vi "Example_BP Network_Classification.vi"() -> ()   [LabVIEW 2020]
uses:
  <vilib>/addons/Machine Learning/Supervised Learning/ml_BP_Terminal Condition.ctl
  <vilib>/Utility/miscctls.llb/LV3DPointTypeDef.ctl
  <vilib>/addons/Machine Learning/Utilities/Training & Test Set (matrix-class).vi
  <vilib>/addons/Machine Learning/Visualization/Visualization (3D).vi
  <vilib>/addons/Machine Learning/NILabs_MLT.lvlib
panel:
  out "Test samples":i32
  in  "Test percentage":dbl
  in  "Num of samples":i32
  out "Lapsed time (ms)":i32
  in  "Data set":enum16{"4 Gaussians", "3 Concentric Circles"}(ring)
  out "Classification accuracy":dbl
  out "Test data":refnum<vi>(3d-picture)
  in  "Stopping criteria":T1={"min MSE"=1e-05, "min delta MSE"=1e-08, "min step length"=1e-08, "max iteration"=1000.0}
  in  "# of hidden neurons":i32=5
  out "Training data":refnum<vi>(3d-picture)
  out "Training MSE":dbl
  # "Introduction:\nA Back-propagation (BP) neural network is applied to two classification problems."
  # "%"
  # "(Samples are overlain with class labels predicted by the BP network.)"
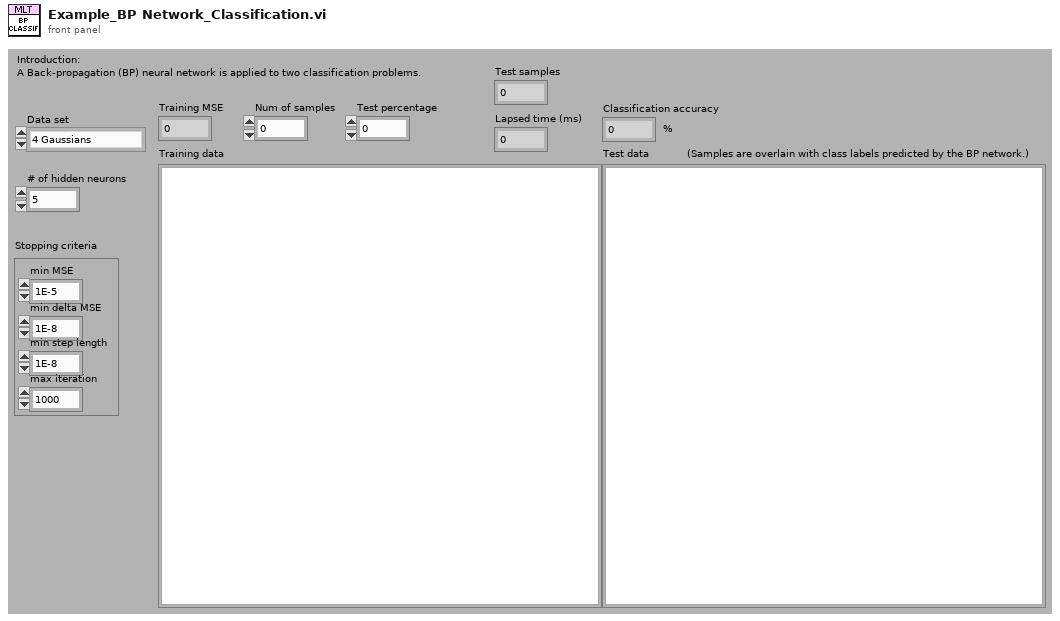
[diagram p1: front panel]
types:
  T1 = typedef "NILabs_MLT.lvlib/ml_BP_Terminal Condition.ctl" = cluster{"min MSE":dbl, "min delta MSE":dbl, "min step length":dbl, "max iteration":dbl}
  T2 = typedef "LV3DPointTypeDef.ctl" = cluster{"X":sgl, "Y":sgl, "Z":sgl}
  T3 = typedef "NILabs_MLT.lvlib/ml_BP_Project.ctl" = cluster{"Training Data":T4, "Normalize Info":T5, "3-layer NN":T6, "Ternimal Condition":T1}
  T4 = typedef "NILabs_MLT.lvlib/ml_BP_Data.ctl" = cluster{"dim in":i32, "dim out":i32, "# samples":i32, "Input":dbl[][], "Output":dbl[][]}
  T5 = typedef "NILabs_MLT.lvlib/ml_BP_Normalize Data.ctl" = cluster{"input min":dbl[], "input max":dbl[], "output min":dbl[], "output max":dbl[]}
  T6 = typedef "NILabs_MLT.lvlib/ml_BP_3layer Feedforward.ctl" = cluster{"# input neuron ":i32, "# hidden neuron":i32, "# output neuron":i32, "Weight (I->H)":dbl[][], "Weight (H->O)":dbl[][], "Output":dbl[][], "Hidden Out":dbl[][], "Derivation Output":dbl[][], "Derivation Hidden":dbl[][], "dw (I->H)":dbl[][], "dw (H->O)":dbl[][]}
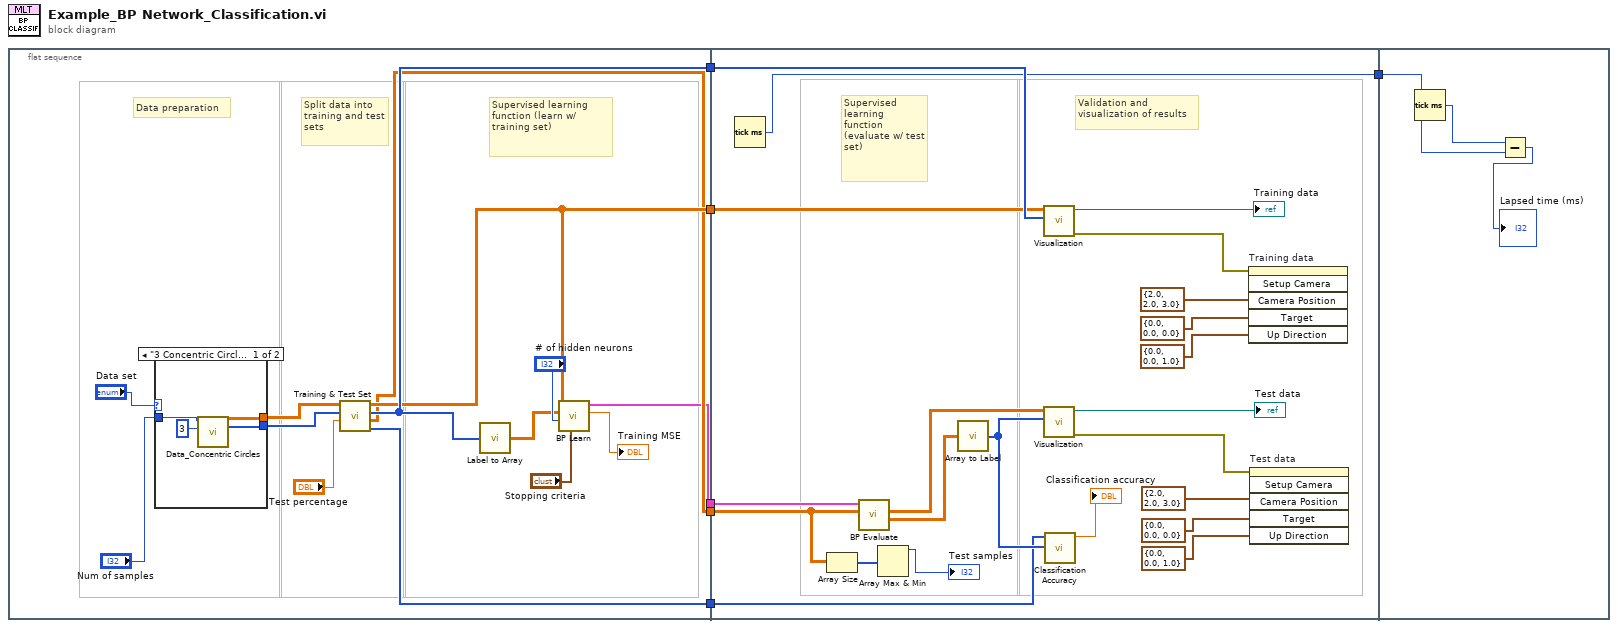
[diagram p0: block diagram]
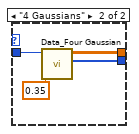
[diagram p2: hidden frame]
diagram:
  n1 = flat-sequence {
    tunnel: [w12] -> w5
    tunnel: [w11] -> w4
    tunnel: [w10] -> w3
    tunnel: [w9] -> w2
    tunnel: [w8] -> w1
    tunnel: [w32] -> w6
    tunnel: w5 -> [w42]
    tunnel: w4 -> [w35]
    tunnel: w3 -> [w34]
    tunnel: w2 -> [w31]
    tunnel: w1 -> [w33]
    tunnel: w6 -> [w53]
    frame #0 {
      # "Supervised learning function (learn w/ training set)"
      # "Split data into training and test sets"
      # "Data preparation"
      n2 = case shown="\"3 Concentric Circles\"" "Data set" {
        tunnel: [w22 w28] -> w20
        tunnel: "Num of samples" -> [w24 w27]
        tunnel: [w21 w26] -> w18
        frame "3 Concentric Circles" {
          n3 = call "Data_Concentric Circles.vi"("# of circles"=3, "# of points"=w24) -> ("Classes"=w21:i32[], "Data"=w22:dbl[][])  [unwired: 8 in]
        }
        frame "4 Gaussians" {
          n4 = call "Data_Four Gaussian.vi"("noise amplitude"=0.35, "# of points"=w27) -> ("Classes"=w26:i32[], "Data"=w28:dbl[][])  [unwired: 8 in]
        }
      }
      n5 = call-poly <vilib>:"Training & Test Set.vi"("percent"="Test percentage", "classes"=w18, "Samples"=w20) -> ("Test Set classes"=w12:i32[], "Test Set Data"=w9:dbl[][], "Training Set classes"=w11:i32[], "Training Set Data"=w10:dbl[][])  [unwired: 5 in]
      n6 = call <vilib>:"Label to Array.vi"("Classes"=w11) -> ("Array"=w17:dbl[][])  [unwired: 1 in]
      n7 = call <vilib>:"BP Learn.vi"("Stopping Criteria"="Stopping criteria", "# of hidden neuron"="# of hidden neurons", "Training outputs"=w17, "Training data samples"=w10) -> ("mse"=→"Training MSE":dbl, "BP Project"=w8:T3)  [unwired: 4 in, 2 out]
    }
    frame #1 {
      # "Validation and visualization of results"
      # "Supervised learning function (evaluate w/ test set)"
      n8 = Tick Count (ms)() -> (millisecond timer value=w32:u32)
      n9 = Array Size(array=w31) -> (size(s)=w30:i32[])
      n10 = call <vilib>:"BP Evaluate.vi"("Test data samples"=w31, "BP Project"=w33) -> ("NN outputs"=w48:dbl[][], "Test data samples dup"=w47:dbl[][])  [unwired: 5 in, 3 out]
      n11 = Array Max & Min(array=w30) -> (max value=→"Test samples":i32)  [unwired: 3 out]
      n12 = call <vilib>:"Array to Label.vi"("Array"=w48) -> ("Classes"=w50:i32[])
      n13 = call-poly <vilib>:"Visualization.vi"("Class labels"=w35, "Data samples"=w34) -> ("error out"=w44:errorcluster, "3D Picture"=→"Training data":refnum<vi>)  [unwired: 8 in]
      n14 = call-poly <vilib>:"Visualization.vi"("Class labels"=w50, "Data samples"=w47) -> ("error out"=w45:errorcluster, "3D Picture"=→"Test data":refnum<vi>)  [unwired: 8 in]
      n15 = call <vilib>:"Classification Accuracy.vi"("Predicted class labels"=w50, "Actual class labels"=w42) -> ("Classification Accuracy"=→"Classification accuracy":dbl)  [unwired: 8 in, 1 out]
      n16 = invoke on="Training data" class="SceneGraphDisp (strict)" method="Setup Camera"(error in=w44, "Camera Position"=T2 {"X"=2.0, "Y"=2.0, "Z"=3.0}, "Target"=T2 {"X"=0.0, "Y"=0.0, "Z"=0.0} ("Camera Position"), "Up Direction"=T2 {"X"=0.0, "Y"=0.0, "Z"=1.0} ("Camera Position")) -> ()  [unwired: 2 in, 6 out]
      n17 = invoke on="Test data" class="SceneGraphDisp (strict)" method="Setup Camera"(error in=w45, "Camera Position"=T2 {"X"=2.0, "Y"=2.0, "Z"=3.0}, "Target"=T2 {"X"=0.0, "Y"=0.0, "Z"=0.0} ("Camera Position"), "Up Direction"=T2 {"X"=0.0, "Y"=0.0, "Z"=1.0} ("Camera Position")) -> ()  [unwired: 2 in, 6 out]
    }
    frame #2 {
      n18 = Tick Count (ms)() -> (millisecond timer value=w52:u32)
      n19 = Subtract(x=w52, y=w53) -> (x-y=→"Lapsed time (ms)":u32)
    }
  }
